vi "SwerveDebugColor.vi"(1 "Azimuth_Angle (deg [-180,180])":dbl, 2 "Drive Velocity (ft/s)":dbl) -> (0 "Color":u32(colorbox))   [LabVIEW 2019]
uses:
  constants.vi
  <vilib>/vision/NI_Vision_Development_Module.lvlib
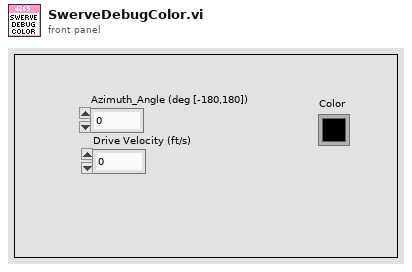
[diagram p1: front panel]
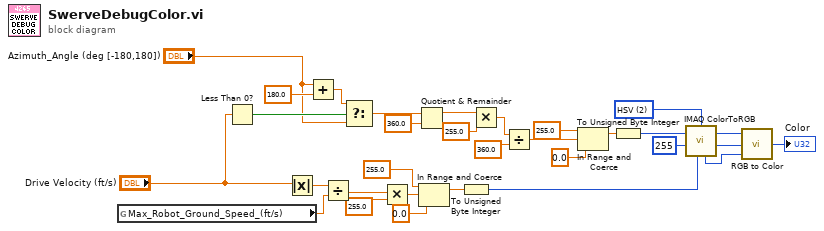
[diagram p0: block diagram]
diagram:
  w31 = u16 2 items=["RGB", "HSL", "HSV", "HSI"] ("Color Mode")
  n1 = global read "constants.vi" "Max_Robot_Ground_Speed_(ft/s)"() -> (w26:dbl)
  n2 = Less Than 0?(x="Drive Velocity (ft/s)") -> (x < 0?=w15:bool)
  n3 = Absolute Value(x="Drive Velocity (ft/s)") -> (abs(x)=w18:dbl)
  n4 = Add(x="Azimuth_Angle (deg [-180,180])", y=180.0) -> (x+y=w13:dbl)
  n5 = Divide(x=w18, y=w26) -> (x/y=w25:dbl)
  n6 = Select(t=w13, s=w15, f="Azimuth_Angle (deg [-180,180])") -> (s? t:f=w12:dbl)
  n7 = Multiply(x=w25, y=255.0) -> (x*y=w23:dbl)
  n8 = Quotient & Remainder(x=w12, y=360.0) -> (x-y*floor(x/y)=w10:dbl)  [unwired: 1 out]
  n9 = In Range and Coerce(upper limit=255.0, x=w23, lower limit=0.0) -> (coerced(x)=w20:dbl)  [unwired: 1 out]
  n10 = To Unsigned Byte Integer(number=w20) -> (unsigned 8bit integer=w19:u8)
  n11 = Multiply(x=w10, y=255.0) -> (x*y=w9:dbl)
  n12 = Divide(x=w9, y=360.0) -> (x/y=w6:dbl)
  n13 = In Range and Coerce(upper limit=255.0, x=w6, lower limit=0.0) -> (coerced(x)=w5:dbl)  [unwired: 1 out]
  n14 = To Unsigned Byte Integer(number=w5) -> (unsigned 8bit integer=w4:u8)
  n15 = call "IMAQ ColorToRGB"("Green or Sat value"=u8 255, "Blue or Luma or Val or Inten value"=w19, "Red or Hue value"=w4, "Color Mode"=w31) -> ("Blue value"=w27:u8, "Green value"=w28:u8, "Red value"=w30:u8)  [unwired: 1 in, 1 out]
  n16 = call <vilib>:"RGB to Color.vi"("B"=w27, "G"=w28, "R"=w30) -> ("Color"=→"Color":u32)
